vi "Details Display Dialog.vi"(0 "Source":string, 1 "Start":i32[](array[numeric]), 2 "Length":i32[](array[numeric]), 3 "code":i32, 4 "Show Link":bool, 5 "Details":string="reason for problem", 7 "dialog type":T3, 9 "Error or Warning":bool, 11 "contname":string="Continue", 12 "stopname":string="Stop", 13 "okname":string="OK", 14 "Tag Found?":T1) -> (15 "stop event propagated":bool)   [LabVIEW 2022 SP3]
uses:
  DialogTypeEnum.ctl
  ErrWarn.ctl
  TagReturnType.ctl
  eventvkey.ctl
panel:
  in  "Search ni.com":bool
  in  "truncated message":string="(source truncated)"
  in  "truncated & CH message":string="(source truncated; see Context Help window)"
  out "Source of Error":string
  out "scrollbar text":string
  in  "Test for size":string
  out "text":string
  out "Error or Warning Glyph":T2=TRUE
  in  "OK":bool
  in  "Stop":bool
  in  "Continue":bool
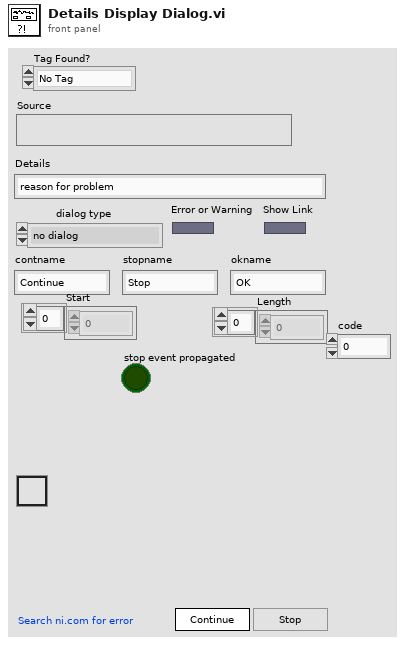
[diagram p1: front panel]
types:
  T1 = typedef "TagReturnType.ctl" = enum16{"No Tag", "<err>", "<append>"}
  T2 = typedef "ErrWarn.ctl" = bool
  T3 = typedef "DialogTypeEnum.ctl" = enum16{"no dialog", "OK message", "continue or stop message", "auto error handling dialog", "OK message + warnings", "continue/stop + warnings"}
  T4 = typedef "eventvkey.ctl" = enum16{"ASCII", "Enter", "Return", "Shift", "Ctrl", "Alt", "Cmd", "Opt", "Caps", "NumLock", "Clear", "Break", "Up", "Down", "Left", "Right", "Insert", "Delete", "Home", "End", "PageUp", "PageDown", "Escape", "Help", "Pause", "ScrollLock", "F1", "F2", "F3", "F4", "F5", "F6", "F7", "F8", "F9", "F10", "F11", "F12", "F13", "F14", "F15", "F16", "F17", "F18", "F19", "F20", "F21", "F22", "F23", "F24", "Play", "VolumeUp", "VolumeDown", "Mute", "Two Byte Char"}
  T5 = enum32{"Invalid", "Standard", "Closed", "Hidden", "Minimized", "Maximized"}
  T6 = typedef "LVRectTypeDef.ctl" = cluster{"Left":i16, "Top":i16, "Right":i16, "Bottom":i16}
  T7 = cluster{"Control":bool, "Shift":bool, "Key":string}
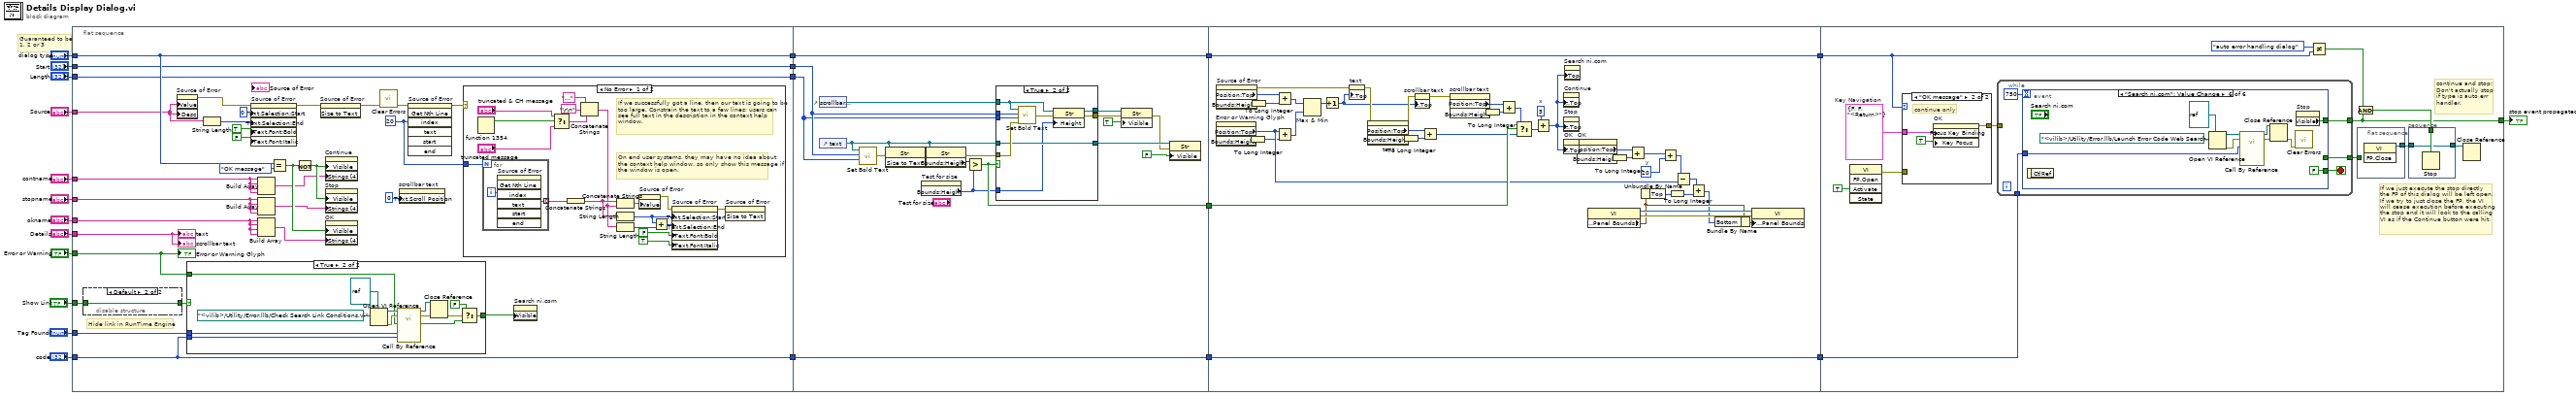
[diagram p0: block diagram]
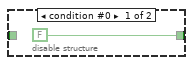
[diagram p2: hidden frame]
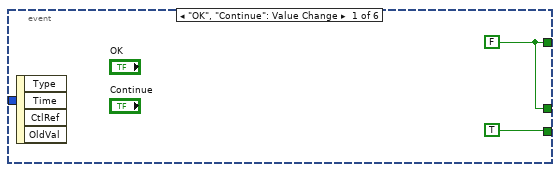
[diagram p6: hidden frame]
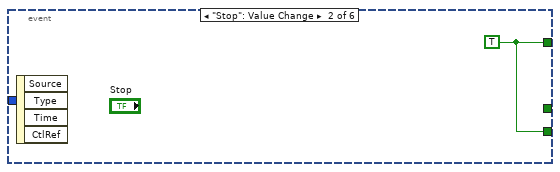
[diagram p7: hidden frame]
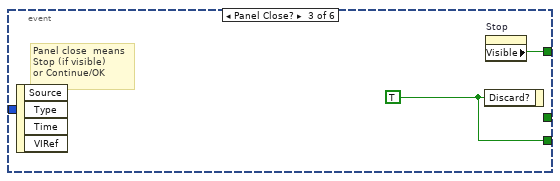
[diagram p8: hidden frame]
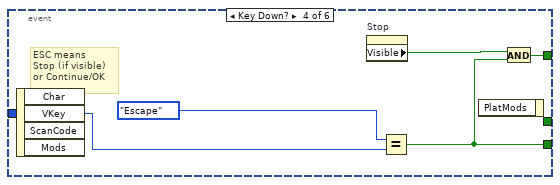
[diagram p9: hidden frame]
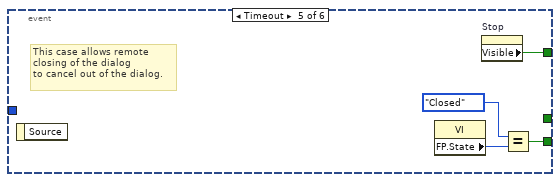
[diagram p10: hidden frame]
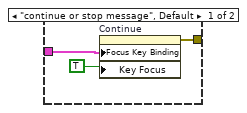
[diagram p11: hidden frame]
diagram:
  # "Guaranteed to be\n1, 2 or 3"
  n1 = flat-sequence {
    tunnel: [w36] -> w21
    tunnel: "dialog type" -> [w36]
    tunnel: "contname" -> [w35]
    tunnel: "stopname" -> [w34]
    tunnel: "okname" -> [w33]
    tunnel: "Source" -> [w29]
    tunnel: "Details" -> [w32]
    tunnel: "Error or Warning" -> [w23]
    tunnel: [w31] -> w10
    tunnel: [w30] -> w9
    tunnel: "Start" -> [w31]
    tunnel: "Length" -> [w30]
    tunnel: "Show Link" -> [w28]
    tunnel: "code" -> [w25]
    tunnel: [w25] -> w2
    tunnel: "Tag Found?" -> [w26]
    tunnel: w21 -> [w92]
    tunnel: [w92] -> w20
    tunnel: [w98] -> w19
    tunnel: w10 -> [w91]
    tunnel: w9 -> [w90]
    tunnel: [w89] -> w3
    tunnel: w2 -> [w89]
    tunnel: w20 -> [w127]
    tunnel: [w127] -> w18
    tunnel: w19 -> [w161]
    tunnel: [w120] -> w4
    tunnel: w3 -> [w120]
    tunnel: [w167] -> w22
    tunnel: w18 -> [w162]
    tunnel: w4 -> [w166]
    frame #0 {
      w43 = u32 20 ("index")
      # "Hide link in RunTime Engine"
      n2 = disable-structure shown="Default" {
        disable-tunnel: w28 -> [_ w55]
        disable-tunnel: [FALSE ("Show Link") w55] -> w27
        frame condition #0 {
        }
        frame condition #1 (active) {
        }
      }
      n3 = property on="Source of Error" class="Str"("Value"=w29, "Desc"=w29) -> (error out=w42:errorcluster)  [unwired: 2 in, 1 out]
      n4 = case shown="True" w27 {
        tunnel: [_ w63] -> w24
        tunnel: w26 -> [_ w62]
        tunnel: w25 -> [_ w61]
        tunnel: w23 -> [_ w60]
        frame False {
        }
        frame True {
          n5 = Open VI Reference(type specifier VI Refnum (for type only)=refnum<vi> refnum, vi path=path "<vilib>/Utility/Error.llb/Check Search Link Conditions.vi") -> (vi reference=w66:refnum<vi>, error out=w68:errorcluster)  [unwired: 4 in]
          n6 = call-by-ref "?"(reference=w66, error in=w68, "Error Code"=w61, "Tag Found?"=w62, "Error or Warning?"=w60) -> (reference out=w59:refnum<vi>, error out=w58:errorcluster, "Display Link?"=w65:bool)  [unwired: 8 in]
          n7 = Close Reference(reference=w59, error in (no error)=w58) -> (error out=w57:errorcluster)
          n8 = Select(t=FALSE, s=w57, f=w65) -> (s? t:f=w63:bool)
        }
      }
      n9 = String Length(string=w29) -> (length=w39:i32)
      n10 = property on="Source of Error" class="Str"(error in=w42, "Text.Selection:Start"=u32 0, "Text.Selection:End"=w39, "Text.Font:Bold"=TRUE, "Text.Font:Italic"=FALSE) -> (error out=w41:errorcluster)  [unwired: 1 in, 1 out]
      n11 = Build Array(w35, w35, w35, w35) -> (w51:string[])
      n12 = Build Array(w34, w34, w34, w34) -> (w50:string[])
      n13 = Build Array(w33, w33, w33, w33) -> (w49:string[])
      n14 = Equal?(x=w36, y=DialogTypeEnum."OK message" ("dialog type")) -> (x = y?=w53:bool)
      n15 = Not(x=w53) -> (.not. x?=w52:bool)
      n16 = invoke on="Source of Error" class="Str" method="Size to Text"(error in=w41) -> (error out=w46:errorcluster)  [unwired: 2 in, 2 out]
      n17 = property on="Continue" class="Bool"("Visible"=w52, "Strings [4]"=w51) -> ()  [unwired: 2 in, 2 out]
      n18 = property on="Stop" class="Bool"("Visible"=w52, "Strings [4]"=w50) -> ()  [unwired: 2 in, 2 out]
      n19 = property on="OK" class="Bool"("Visible"=w53, "Strings [4]"=w49) -> ()  [unwired: 2 in, 2 out]
      n20 = call "Clear Errors.vi"("error in (no error)"=w46) -> ("error out"=w45:errorcluster)  [unwired: 5 in, 1 out]
      n21 = property on="scrollbar text" class="Str"("Text.Scroll Position"=u32 0) -> ()  [unwired: 2 in, 2 out]
      n22 = invoke on="Source of Error" class="Str" method="Get Nth Line"(error in=w45, "index"=w43) -> (error out=w44:errorcluster)  [unwired: 5 in, 6 out]
      n23 = case shown="No Error" w44 {
        tunnel: w43 -> [w86 _]
        frame No Error {
          # "If we successfully got a line, then our text is going to be too large. Constrain the text to a few lines; users can see full text in the description in the context help window."
          # "On end user systems, they may have no idea about\nthe context help window, so only show this message if\nthe window is open."
          n24 = fn#1354() -> (1:w76:bool)  [unwired: 1 out]
          n25 = for {
            N: w86 -> [_]
            tunnel: [w87] -> w84 mode=indexing
            i -> [w88]
            n26 = invoke on="Source of Error" class="Str" method="Get Nth Line"("index"=w88) -> ("text"=w87:string)  [unwired: 6 in, 6 out]
          }
          n27 = Select(t="truncated & CH message", s=w76, f="truncated message") -> (s? t:f=w73:string)
          n28 = Concatenate Strings(w84) -> (w83:string)
          n29 = Concatenate Strings("..." ("string"), "\r\n", w73) -> (w70:string)
          n30 = Concatenate Strings(w83, w70) -> (w85:string)
          n31 = String Length(string=w83) -> (length=w78:i32)
          n32 = String Length(string=w70) -> (length=w75:i32)
          n33 = property on="Source of Error" class="Str"("Value"=w85) -> (error out=w80:errorcluster)  [unwired: 2 in, 1 out]
          n34 = Add(x=w78, y=w75) -> (x+y=w77:i32)
          n35 = property on="Source of Error" class="Str"(error in=w80, "Text.Selection:Start"=w78, "Text.Selection:End"=w77, "Text.Font:Bold"=FALSE, "Text.Font:Italic"=TRUE) -> (error out=w79:errorcluster)  [unwired: 1 in, 1 out]
          n36 = invoke on="Source of Error" class="Str" method="Size to Text"(error in=w79) -> ()  [unwired: 2 in, 3 out]
        }
        frame Error {
          # "An error at this point means that there is no line to fetch. That's good. We do not want the text getting too large."
        }
      }
      n37 = property on="Search ni.com" class="Bool"("Visible"=w24) -> ()  [unwired: 2 in, 2 out]
      "Error or Warning Glyph" <- w23
      "scrollbar text" <- w32
      "text" <- w32
    }
    frame #1 {
      n38 = control-ref of="scrollbar text"() -> (w101:refnum<vi>)
      n39 = control-ref of="text"() -> (w93:refnum<vi>)
      n40 = call "Set Bold Text.vi"("Length"=w90, "Start"=w91, "text"=w93) -> ("error out"=w96:errorcluster)  [unwired: 3 in]
      n41 = invoke class="Str" method="Size to Text"(reference=w93, error in=w96) -> (error out=w97:errorcluster)  [unwired: 1 in, 2 out]
      n42 = property on="Test for size" class="Str"() -> ("Bounds:Height"=w95:u32)  [unwired: 2 in, 2 out]
      n43 = property class="Str"(reference=w93, error in=w97) -> (error out=w105:errorcluster, "Bounds:Height"=w106:u32)  [unwired: 1 out]
      n44 = Greater?(x=w106, y=w95) -> (0:w98:bool)
      n45 = case shown="True" w98 {
        tunnel: w105 -> [w109 w118]
        tunnel: w91 -> [_ w117]
        tunnel: w90 -> [_ w116]
        tunnel: [w109 w113] -> w94
        tunnel: w93 -> [w108 w115]
        tunnel: [w108 w110] -> w103
        tunnel: [w107 w115] -> w102
        tunnel: w101 -> [w107 w111]
        tunnel: w95 -> [_ w114]
        frame False {
        }
        frame True {
          n46 = call "Set Bold Text.vi"("error in"=w118, "Length"=w116, "Start"=w117, "text"=w111) -> ("error out"=w112:errorcluster)  [unwired: 2 in]
          n47 = property class="Str"(reference=w111, error in=w112, "Height"=w114) -> (reference out=w110:refnum<vi>, error out=w113:errorcluster)
        }
      }
      n48 = property class="Str"(reference=w103, error in=w94, "Visible"=TRUE ("Defer Panel Updates")) -> (error out=w99:errorcluster)  [unwired: 1 out]
      n49 = property class="Str"(reference=w102, error in=w99, "Visible"=FALSE ("Defer Panel Updates")) -> ()  [unwired: 2 out]
    }
    frame #2 {
      w148 = 20  # y
      w153 = 5  # x
      n50 = property on="Error or Warning Glyph" class="Bool"() -> ("Position:Top"=w143:i32, "Bounds:Height"=w158:u32)  [unwired: 2 in, 2 out]
      n51 = property on="Source of Error" class="Str"() -> (error out=w128:errorcluster, "Position:Top"=w130:i32, "Bounds:Height"=w129:u32)  [unwired: 2 in, 1 out]
      n52 = To Long Integer(number=w158) -> (32bit integer=w126:i32)
      n53 = To Long Integer(number=w129) -> (32bit integer=w125:i32)
      n54 = Add(x=w130, y=w125) -> (x+y=w160:i32)
      n55 = Add(x=w143, y=w126) -> (x+y=w159:i32)
      n56 = Max & Min(x=w160, y=w159) -> (max(x,y)=w157:i32)  [unwired: 1 out]
      n57 = Increment(x=w157) -> (x+1=w136:i32)
      n58 = property on="text" class="Str"(error in=w128, "Position:Top"=w136) -> (error out=w138:errorcluster)  [unwired: 1 in, 1 out]
      n59 = property on="text" class="Str"(error in=w138) -> (error out=w137:errorcluster, "Position:Top"=w135:i32, "Bounds:Height"=w134:u32)  [unwired: 1 in, 1 out]
      n60 = To Long Integer(number=w134) -> (32bit integer=w124:i32)
      n61 = property on="scrollbar text" class="Str"(error in=w137, "Position:Top"=w136) -> (error out=w156:errorcluster)  [unwired: 1 in, 1 out]
      n62 = Add(x=w135, y=w124) -> (x+y=w132:i32)
      n63 = property on="scrollbar text" class="Str"(error in=w156) -> ("Position:Top"=w155:i32, "Bounds:Height"=w154:u32)  [unwired: 1 in, 2 out]
      n64 = To Long Integer(number=w154) -> (32bit integer=w123:i32)
      n65 = Add(x=w155, y=w123) -> (x+y=w133:i32)
      n66 = Select(t=w133, s=w161, f=w132) -> (s? t:f=w131:i32)
      n67 = Add(x=w153, y=w131) -> (x+y=w119:i32)
      n68 = property on="Continue" class="Bool"("Position:Top"=w119) -> ()  [unwired: 2 in, 2 out]
      n69 = property on="Stop" class="Bool"("Position:Top"=w119) -> ()  [unwired: 2 in, 2 out]
      n70 = property on="OK" class="Bool"("Position:Top"=w119) -> (error out=w152:errorcluster)  [unwired: 2 in, 1 out]
      n71 = property on="Search ni.com" class="Bool"("Top"=w119) -> ()  [unwired: 2 in, 2 out]
      n72 = property on="OK" class="Bool"(error in=w152) -> ("Position:Top"=w150:i32, "Bounds:Height"=w151:u32)  [unwired: 1 in, 2 out]
      n73 = property class="VI"() -> (reference out=w145:refnum<vi>, error out=w146:errorcluster, "Front Panel Window:Panel Bounds"=w142:T6)  [unwired: 2 in]
      n74 = To Long Integer(number=w151) -> (32bit integer=w122:i32)
      n75 = Add(x=w150, y=w122) -> (x+y=w149:i32)
      n76 = Unbundle By Name(w142) -> ("Top"=w140:i16)
      n77 = Add(x=w149, y=w148) -> (x+y=w144:i32)
      n78 = To Long Integer(number=w140) -> (32bit integer=w121:i32)
      n79 = Subtract(x=w144, y=w143) -> (x-y=w141:i32)
      n80 = Add(x=w141, y=w121) -> (x+y=w139:i32)
      n81 = Bundle By Name(cluster=w142, "Bottom"=w139) -> (w147:T6)
      n82 = property class="VI"(reference=w145, error in=w146, "Front Panel Window:Panel Bounds"=w147) -> ()  [unwired: 2 out]
    }
    frame #3 {
      w174 = T7 {"Control"=FALSE, "Shift"=FALSE, "Key"="<Return>"}  # Key Navigation
      # "If we just execute the stop directly\nthe FP of this dialog will be left open.\nIf we try to just close the FP, the VI\nwill cease execution before executing\nthe stop and it will look to the calling\nVI as if the Continue button were hit."
      # "continue and stop;\nDon't actually stop\nif type is auto err\nhandler."
      n83 = invoke class="VI" method="FP.Open"("Activate"=TRUE ("Front Panel Window:Open")) -> (error out=w164:errorcluster)  [unwired: 4 in, 4 out]
      n84 = case shown="\"OK message\"" w162 {
        tunnel: w174 -> [w209 w212]
        tunnel: w164 -> [_ _]
        tunnel: [w207 w210] -> w173
        frame "continue or stop message", Default {
          n85 = property on="Continue" class="Bool"("Focus Key Binding"=w209, "Key Focus"=TRUE) -> (error out=w207:errorcluster)  [unwired: 2 in, 1 out]
        }
        frame "OK message" {
          # "continue only"
          n86 = property on="OK" class="Bool"("Focus Key Binding"=w212, "Key Focus"=TRUE) -> (error out=w210:errorcluster)  [unwired: 2 in, 1 out]
        }
      }
      n87 = while {
        tunnel: w173 -> [_]
        tunnel: [w181] -> w167
        tunnel: [w180] -> w163
        tunnel: w166 -> [w178]
        stop <- w182 stop-if-true
        n88 = event shown="[5] \"Search ni.com\": Value Change" {
          selector: _ -> [_ _ _ _ _ _]
          dyn-events: _ -> [_ _ _ _ _ _]
          timeout: 750 -> [_ _ _ _ _ _]
          tunnel: [TRUE ("Stop") w185 w187 w188 w194 FALSE ("Discard?")] -> w182
          tunnel: [w184 w185 w186 w191 w196 w206] -> w181
          tunnel: [w184 _ _ _ _ _] -> w180
          tunnel: w178 -> [_ _ _ _ _ w201]
          event "OK", "Continue": Value Change {
            w184 = FALSE ("Stop")
            n89 = event-data() -> ()  [unwired: 1 in, 4 out]
          }
          event "Stop": Value Change {
            w185 = TRUE
            n90 = event-data() -> ()  [unwired: 1 in, 4 out]
          }
          event Panel Close? {
            w187 = TRUE ("Discard?")
            # "Panel close  means\nStop (if visible)\nor Continue/OK"
            n91 = event-data() -> ()  [unwired: 1 in, 4 out]
            n92 = event-data("Discard?"=w187) -> ()  [unwired: 1 in, 1 out]
            n93 = property on="Stop" class="Bool"() -> ("Visible"=w186:bool)  [unwired: 2 in, 2 out]
          }
          event Key Down? {
            # "ESC means\nStop (if visible)\nor Continue/OK"
            n94 = event-data() -> ("VKey"=w190:T4)  [unwired: 1 in, 3 out]
            n95 = property on="Stop" class="Bool"() -> ("Visible"=w192:bool)  [unwired: 2 in, 2 out]
            n96 = Equal?(x=eventvkey."Escape", y=w190) -> (x = y?=w188:bool)
            n97 = event-data() -> ()  [unwired: 2 in, 1 out]
            n98 = And(x=w192, y=w188) -> (x .and. y?=w191:bool)
          }
          event Timeout {
            # "This case allows remote\nclosing of the dialog\nto cancel out of the dialog."
            n99 = event-data() -> ()  [unwired: 1 in, 1 out]
            n100 = property class="VI"() -> ("FP.State"=w195:T5)  [unwired: 2 in, 2 out]
            n101 = property on="Stop" class="Bool"() -> ("Visible"=w196:bool)  [unwired: 2 in, 2 out]
            n102 = Equal?(x=T5."Closed", y=w195) -> (x = y?=w194:bool)
          }
          event "Search ni.com": Value Change {
            n103 = event-data() -> ()  [unwired: 1 in, 1 out]
            n104 = Open VI Reference(type specifier VI Refnum (for type only)=refnum<vi> refnum, vi path=path "<vilib>/Utility/Error.llb/Launch Error Code Web Search.vi") -> (vi reference=w204:refnum<vi>, error out=w202:errorcluster)  [unwired: 4 in]
            n105 = call-by-ref "?"(reference=w204, error in=w202, "Code"=w201) -> (reference out=w200:refnum<vi>, error out=w199:errorcluster)  [unwired: 11 in]
            n106 = Close Reference(reference=w200, error in (no error)=w199) -> (error out=w198:errorcluster)
            n107 = call "Clear Errors.vi"("error in (no error)"=w198) -> ()  [unwired: 5 in, 2 out]
            n108 = property on="Stop" class="Bool"() -> ("Visible"=w206:bool)  [unwired: 2 in, 2 out]
          }
        }
      }
      n109 = Not Equal?(x=DialogTypeEnum."auto error handling dialog" ("dialog type"), y=w162) -> (x != y?=w172:bool)
      n110 = flat-sequence {
        tunnel: [w175] -> w169
        tunnel: w163 -> [_]
        frame #0 {
          n111 = invoke class="VI" method="FP.Close"() -> (reference out=w175:refnum<vi>)  [unwired: 3 in, 2 out]
        }
      }
      n112 = And(x=w172, y=w167) -> (x .and. y?=w171:bool)
      n113 = stacked-sequence {
        tunnel: w169 -> [w176]
        tunnel: w171 -> [w177]
        tunnel: [w176] -> w170
        frame #0 {
          n114 = Stop(stop? (T)=w177) -> ()
        }
      }
      n115 = Close Reference(reference=w170) -> ()  [unwired: 1 in, 1 out]
    }
  }
  "stop event propagated" <- w22
